vi "BuildExperiment.vi"(0 "object in":refnum<class "Experiment.lvclass">, 1 "List of Frequencies":dbl[](array[numeric]) min=0.001, 2 "List of Powers to run(W)":dbl[](array[numeric]) min=0.001, 3 "Number of Images":i32, 4 "wait time(s)":dbl, 5 "error in (no error)":errorcluster, 6 "AutoRange MSO":bool, 7 "Flow":dbl[](array[numeric]), 8 "wait after changing flow rate(s)":dbl, 9 "Repeat Adjust Power and Wait N Times":i32, 11 "wait after adjust power":dbl) -> (14 "object out":refnum<class "Experiment.lvclass">, 17 "# elements in queue":i32, 19 "error out":errorcluster)   [LabVIEW 2023, in "Experiment.lvclass"]
uses:
  Experiment.lvclass
  Experiment.lvclass/Experiment.ctl
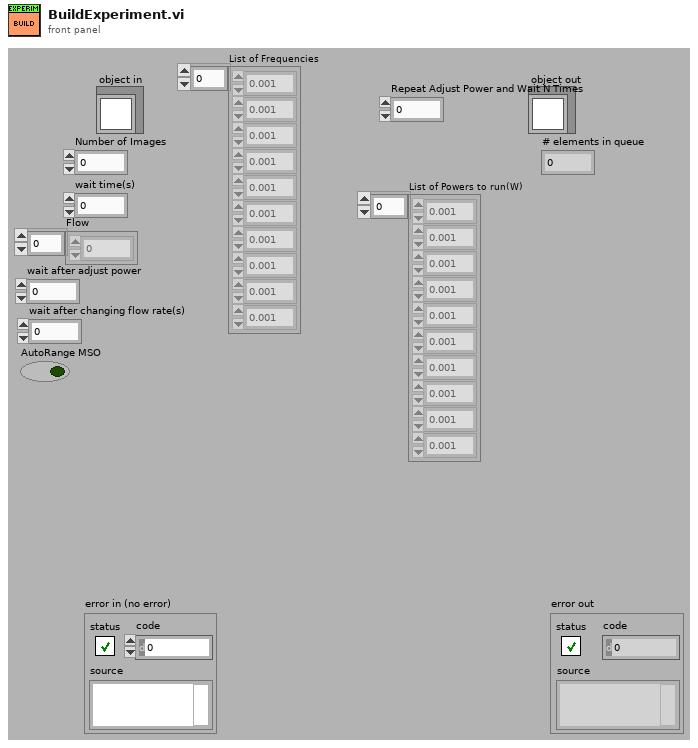
[diagram p1: front panel]
types:
  T1 = cluster{"index":i32, "Level(ml)":dbl, "Flow":dbl}
  T2 = cluster{"Enable Output WFG Ch1":bool, "Enable Output WFG Ch 2":bool}
  T3 = cluster{"Ch1.Carrier.Frequency (Hz)":dbl, "Ch2.Carrier.Frequency (Hz)":dbl}
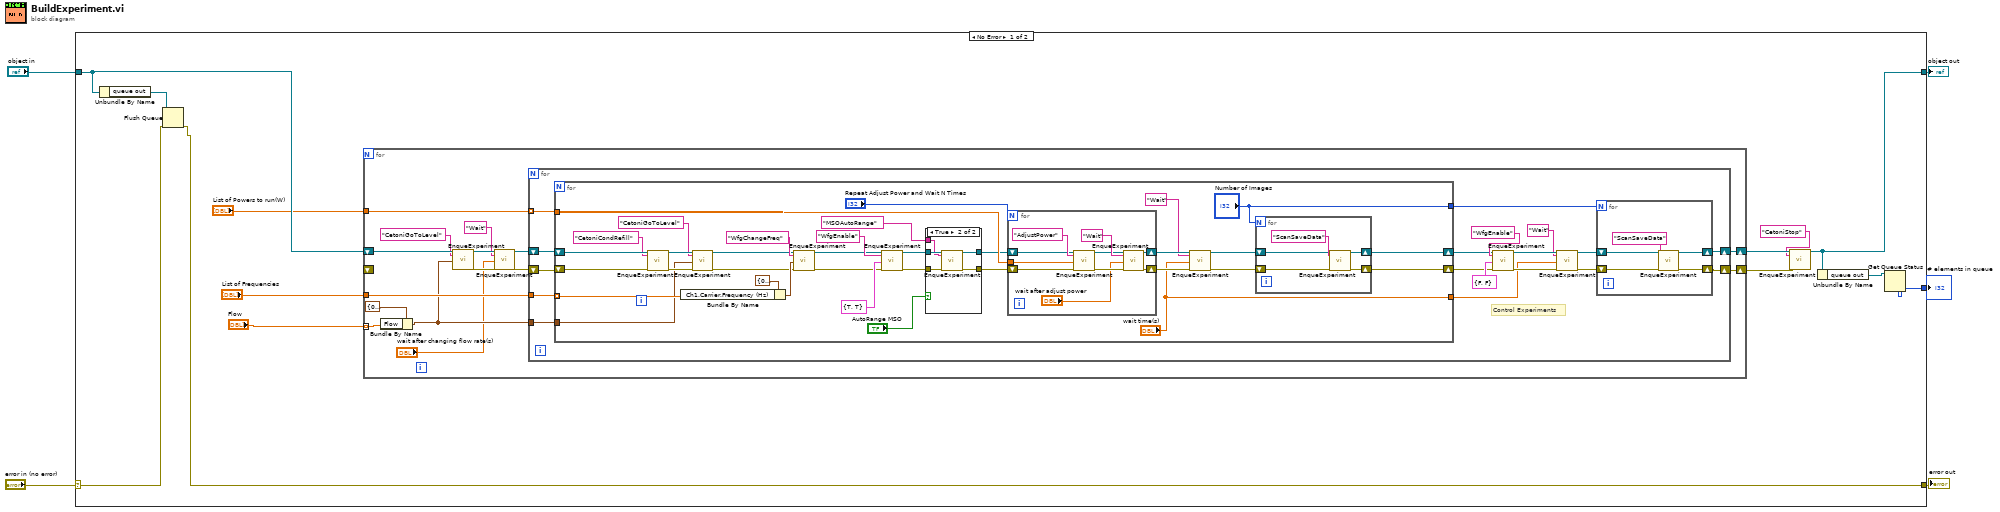
[diagram p0: block diagram]
diagram:
  n1 = case shown="No Error" "error in (no error)" {
    selector: "error in (no error)" -> [w15 w114]
    tunnel: [w14 w114] -> w4
    tunnel: [w8 w113] -> w2
    tunnel: "object in" -> [w17 w113]
    tunnel: [w12 _] -> w1
    frame No Error {
      n2 = Unbundle By Name(w17) -> ("queue out"=w16:refnum<queue>)
      n3 = Flush Queue(queue=w16, error in (no error)=w15) -> (error out=w14:errorcluster)  [unwired: 2 out]
      n4 = for {
        tunnel: "List of Frequencies" -> [w33]
        tunnel: "List of Powers to run(W)" -> [w31]
        shift-right: [w32] -> w9
        shift-left: w17 -> [w27]
        shift-right: [w30] -> w7
        shift-left: _ -> [_]
        tunnel: "Flow" -> [w28] mode=indexing
        n5 = Bundle By Name(cluster=T1 {"index"=0, "Level(ml)"=0.0, "Flow"=0.0} ("GoToLevelSettings"), "Flow"=w28) -> (w26:T1)
        n6 = call-dynamic "EnqueExperiment.vi"("object in"=w27, "Message"="CetoniGoToLevel", "Message Data"=w26) -> ("object out"=w24:refnum<class "Experiment.lvclass">, "error out"=w22:errorcluster)  [unwired: 15 in]
        n7 = call-dynamic "EnqueExperiment.vi"("object in"=w24, "Message"="Wait", "Message Data"="wait after changing flow rate(s)", "error in (no error)"=w22) -> ("object out"=w23:refnum<class "Experiment.lvclass">, "error out"=w21:errorcluster)  [unwired: 14 in]
        n8 = for {
          tunnel: w33 -> [w50]
          shift-right: [w41] -> w32
          shift-left: w23 -> [w49]
          tunnel: w31 -> [w51] mode=indexing
          tunnel: w26 -> [w35]
          shift-right: [w36] -> w30
          shift-left: w21 -> [w34]
          # "Control Experiments"
          n9 = for {
            tunnel: w51 -> [w90]
            shift-right: [w80] -> w40
            shift-left: w49 -> [w78]
            tunnel: w50 -> [w83] mode=indexing
            tunnel: ["Number of Images"] -> w37
            shift-right: [w79] -> w38
            shift-left: w34 -> [w77]
            tunnel: ["wait time(s)"] -> w39
            tunnel: w35 -> [w71]
            n10 = call-dynamic "EnqueExperiment.vi"("object in"=w78, "Message"="CetoniCondRefill", "error in (no error)"=w77) -> ("object out"=w73:refnum<class "Experiment.lvclass">, "error out"=w75:errorcluster)  [unwired: 15 in]
            n11 = Bundle By Name(cluster=T3 {"Ch1.Carrier.Frequency (Hz)"=0.0, "Ch2.Carrier.Frequency (Hz)"=0.0} ("Freq Ch1&2"), "Ch1.Carrier.Frequency (Hz)"=w83) -> (w84:T3)
            n12 = call-dynamic "EnqueExperiment.vi"("object in"=w73, "Message"="CetoniGoToLevel", "Message Data"=w71, "error in (no error)"=w75) -> ("object out"=w72:refnum<class "Experiment.lvclass">, "error out"=w74:errorcluster)  [unwired: 14 in]
            n13 = call-dynamic "EnqueExperiment.vi"("object in"=w72, "Message"="WfgChangeFreq", "Message Data"=w84, "error in (no error)"=w74) -> ("object out"=w87:refnum<class "Experiment.lvclass">, "error out"=w82:errorcluster)  [unwired: 14 in]
            n14 = call-dynamic "EnqueExperiment.vi"("object in"=w87, "Message"="WfgEnable", "Message Data"=T2 {"Enable Output WFG Ch1"=TRUE, "Enable Output WFG Ch 2"=TRUE} ("OutputEnable 2"), "error in (no error)"=w82) -> ("object out"=w62:refnum<class "Experiment.lvclass">, "error out"=w60:errorcluster)  [unwired: 14 in]
            n15 = case shown="True" "AutoRange MSO" {
              tunnel: w62 -> [w92 w97]
              tunnel: [w92 w96] -> w61
              tunnel: w60 -> [w91 w95]
              tunnel: [w91 w94] -> w59
              tunnel: "MSOAutoRange" ("Message") -> [_ w93]
              frame False {
              }
              frame True {
                n16 = call-dynamic "EnqueExperiment.vi"("object in"=w97, "Message"=w93, "error in (no error)"=w95) -> ("object out"=w96:refnum<class "Experiment.lvclass">, "error out"=w94:errorcluster)  [unwired: 15 in]
              }
            }
            n17 = for {
              N: "Repeat Adjust Power and Wait N Times" -> [_]
              tunnel: w90 -> [w107]
              shift-right: [w101] -> w68
              shift-left: w61 -> [w100]
              shift-right: [w103] -> w66
              shift-left: w59 -> [w99]
              n18 = call-dynamic "EnqueExperiment.vi"("object in"=w100, "Message"="AdjustPower", "Message Data"=w107, "error in (no error)"=w99) -> ("object out"=w102:refnum<class "Experiment.lvclass">, "error out"=w104:errorcluster)  [unwired: 14 in]
              n19 = call-dynamic "EnqueExperiment.vi"("object in"=w102, "Message"="Wait", "Message Data"="wait after adjust power", "error in (no error)"=w104) -> ("object out"=w101:refnum<class "Experiment.lvclass">, "error out"=w103:errorcluster)  [unwired: 14 in]
            }
            n20 = call-dynamic "EnqueExperiment.vi"("object in"=w68, "Message"="Wait", "Message Data"="wait time(s)", "error in (no error)"=w66) -> ("object out"=w67:refnum<class "Experiment.lvclass">, "error out"=w65:errorcluster)  [unwired: 14 in]
            n21 = for {
              N: "Number of Images" -> [_]
              shift-right: [w109] -> w80
              shift-left: w67 -> [w110]
              shift-right: [w108] -> w79
              shift-left: w65 -> [w111]
              n22 = call-dynamic "EnqueExperiment.vi"("object in"=w110, "Message"="ScanSaveData", "error in (no error)"=w111) -> ("object out"=w109:refnum<class "Experiment.lvclass">, "error out"=w108:errorcluster)  [unwired: 15 in]
            }
          }
          n23 = call-dynamic "EnqueExperiment.vi"("object in"=w40, "Message"="WfgEnable", "Message Data"=T2 {"Enable Output WFG Ch1"=FALSE, "Enable Output WFG Ch 2"=FALSE} ("OutputEnable 2"), "error in (no error)"=w38) -> ("object out"=w45:refnum<class "Experiment.lvclass">, "error out"=w47:errorcluster)  [unwired: 14 in]
          n24 = call-dynamic "EnqueExperiment.vi"("object in"=w45, "Message"="Wait", "Message Data"=w39, "error in (no error)"=w47) -> ("object out"=w46:refnum<class "Experiment.lvclass">, "error out"=w48:errorcluster)  [unwired: 14 in]
          n25 = for {
            N: w37 -> [_]
            shift-right: [w53] -> w36
            shift-left: w48 -> [w55]
            shift-right: [w52] -> w41
            shift-left: w46 -> [w54]
            n26 = call-dynamic "EnqueExperiment.vi"("object in"=w54, "Message"="ScanSaveData", "error in (no error)"=w55) -> ("object out"=w52:refnum<class "Experiment.lvclass">, "error out"=w53:errorcluster)  [unwired: 15 in]
          }
        }
      }
      n27 = call-dynamic "EnqueExperiment.vi"("object in"=w9, "Message"="CetoniStop", "error in (no error)"=w7) -> ("object out"=w8:refnum<class "Experiment.lvclass">)  [unwired: 15 in, 1 out]
      n28 = Unbundle By Name(w8) -> ("queue out"=w13:refnum<queue>)
      n29 = Get Queue Status(queue=w13) -> (# elements in queue=w12:i32)  [unwired: 2 in, 7 out]
    }
    frame Error {
    }
  }
  "error out" <- w4
  "object out" <- w2
  "# elements in queue" <- w1
